vi "Main.vi"(11 "Module Admin":refnum<class "Delacor_lib_QMH_Module Admin.lvclass">) -> ()   [LabVIEW 2021, in "Master.lvlib"]
doc: "This template is based off of the Queued Message Handler design pattern and the Queued Message Handler project template that ships with LabVIEW.\n\nThe main difference is that the queue is private to this module and communication between modules is performed via Broadcast and Request events.\n\nRequest events are wrapped in public API methods and are handled in the Event Handling Loop (EHL) of this VI. Any module can register for Broadcast events sent by this module. The EHL generates messages based on user interface actions.\n\nThe Message Handling Loop (MHL) processes messages generated by the EHL, or by other messages. The messages are string values, so new messages can be added easily to the Message Cases case structure in the MHL. Each message cluster can also provide an optional value for Message Data, which is a variant that can be converted to whatever message-specific data is required.\n_____\nBased on DQMH Project Template 6.1.0.94.\n\n<b>Note:</b> This VI was modified by the <b>Validate DQMH Module</b> tool to add a 'Panel Hidden' status updated broadcast to the Panel Close? event when External Launch = TRUE.\n\n<b>Note:</b> This VI was modified by the <b>Validate DQMH Module</b> tool to add a call to the Error Reported VI at the end of the 'Exit' MHL frame.\n\n<b>Note:</b> This VI was modified by the <b>Validate DQMH Module</b> tool to wrap the FP.Open method in the module close code with a Conditional Disable Structure so it does not execute when the Main VI is running as a built EXE."
uses:
  Master.lvlib
  <vilib>/Delacor/Delacor QMH/Libraries/Module Admin_class/Delacor_lib_QMH_Module Admin.lvclass
  Custom/class Master/Master.lvclass
  <vilib>/Delacor/Delacor QMH/Libraries/Message Queue_class/Delacor_lib_QMH_Message Queue.lvclass/Delacor_lib_QMH_Message Queue.ctl
  Stop Argument--cluster.ctl
  <vilib>/Delacor/Delacor QMH/Libraries/Module Admin_class/Delacor_lib_QMH_Module Admin.lvclass/Delacor_lib_QMH_Module Admin.ctl
  Slave Stop Argument--cluster.ctl
  <vilib>/Utility/miscctls.llb/LVPointTypeDef.ctl
  Slave Launch Argument--cluster.ctl
  <vilib>/Delacor/Delacor QMH/Libraries/Message Queue_class/Delacor_lib_QMH_Enqueue Message (Single).vi
  <vilib>/Delacor/Delacor QMH/Libraries/Module Admin_class/Delacor_lib_QMH_Get External Launch.vi
  <vilib>/Utility/error.llb/Error Cluster From Error Code.vi
  <vilib>/ErrorRing/Error Ring.xnode
  <vilib>/Delacor/Delacor QMH/Libraries/Message Queue_class/Delacor_lib_QMH_Message Queue.lvclass
  Slave/Slave.lvlib
panel:
  in  "Slaves":i32=2
  in  "Launch Array":bool
  in  "Show Hide":bool
  out "Slave Launched":i32
  out "Slave Init":i32
  out "Slave Init?":bool
  in  "Show Slave":bool
  out "Err Module ID":i32
  out "Additional Information":string
  out "Slaves Error":errorcluster
  in  "Module ID":i32
  out "Slave IDs":i32[](array[numeric])
  in  "Stop Slave":bool
  in  "Launch Slave":bool
  out "Title":string
  out "error out":errorcluster
  out "Status":string
  in  "Simulate MHL Error":bool
  in  "Simulate EHL Error":bool
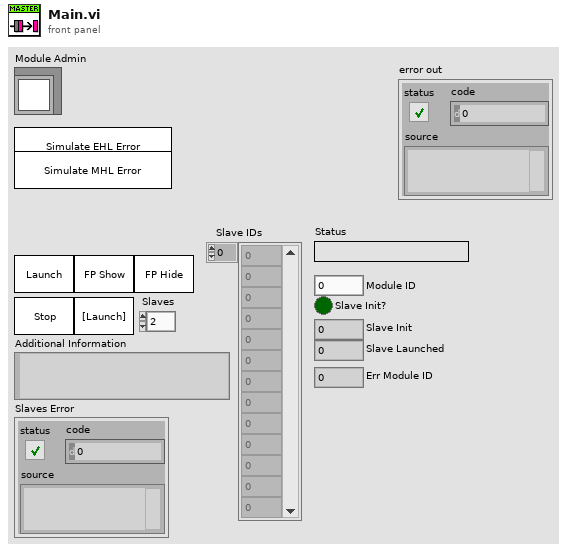
[diagram p1: front panel]
types:
  T1 = typedef "Master.lvlib/Request Events--cluster.ctl" = cluster{"Stop Module":refnum<user-event>, "Show Panel":refnum<user-event>, "Hide Panel":refnum<user-event>, "Get Module Execution Status":refnum<user-event>, "Show Diagram":refnum<user-event>, "Slave Launch":refnum<user-event>, "Slave Stop":refnum<user-event>}
  T2 = typedef "Slave.lvlib/Broadcast Events--cluster.ctl" = cluster{"Module Did Init":refnum<user-event>, "Status Updated":refnum<user-event>, "Error Reported":refnum<user-event>, "Module Did Stop":refnum<user-event>, "Update Module Execution Status":refnum<user-event>}
  T3 = enum32{"invalid lock state", "Not Locked", "Locked (No Password)", "Password-protected"}
  T4 = typedef "Master.lvlib/Stop Argument--cluster.ctl" = cluster{"Origin":string, "Exit via Stop Module Req?":bool, "Wait for Module to stop?":bool}
  T5 = typedef "Master.lvlib/Slave Stop Argument--cluster.ctl" = cluster{"Module ID":i32}
  T6 = typedef "LVPointTypeDef.ctl" = cluster{"Horizontal":i16, "Vertical":i16}
  T7 = enum32{"Invalid", "Standard", "Closed", "Hidden", "Minimized", "Maximized"}
  T8 = typedef "Master.lvlib/Slave Launch Argument--cluster.ctl" = cluster{"ModuleID":i32}
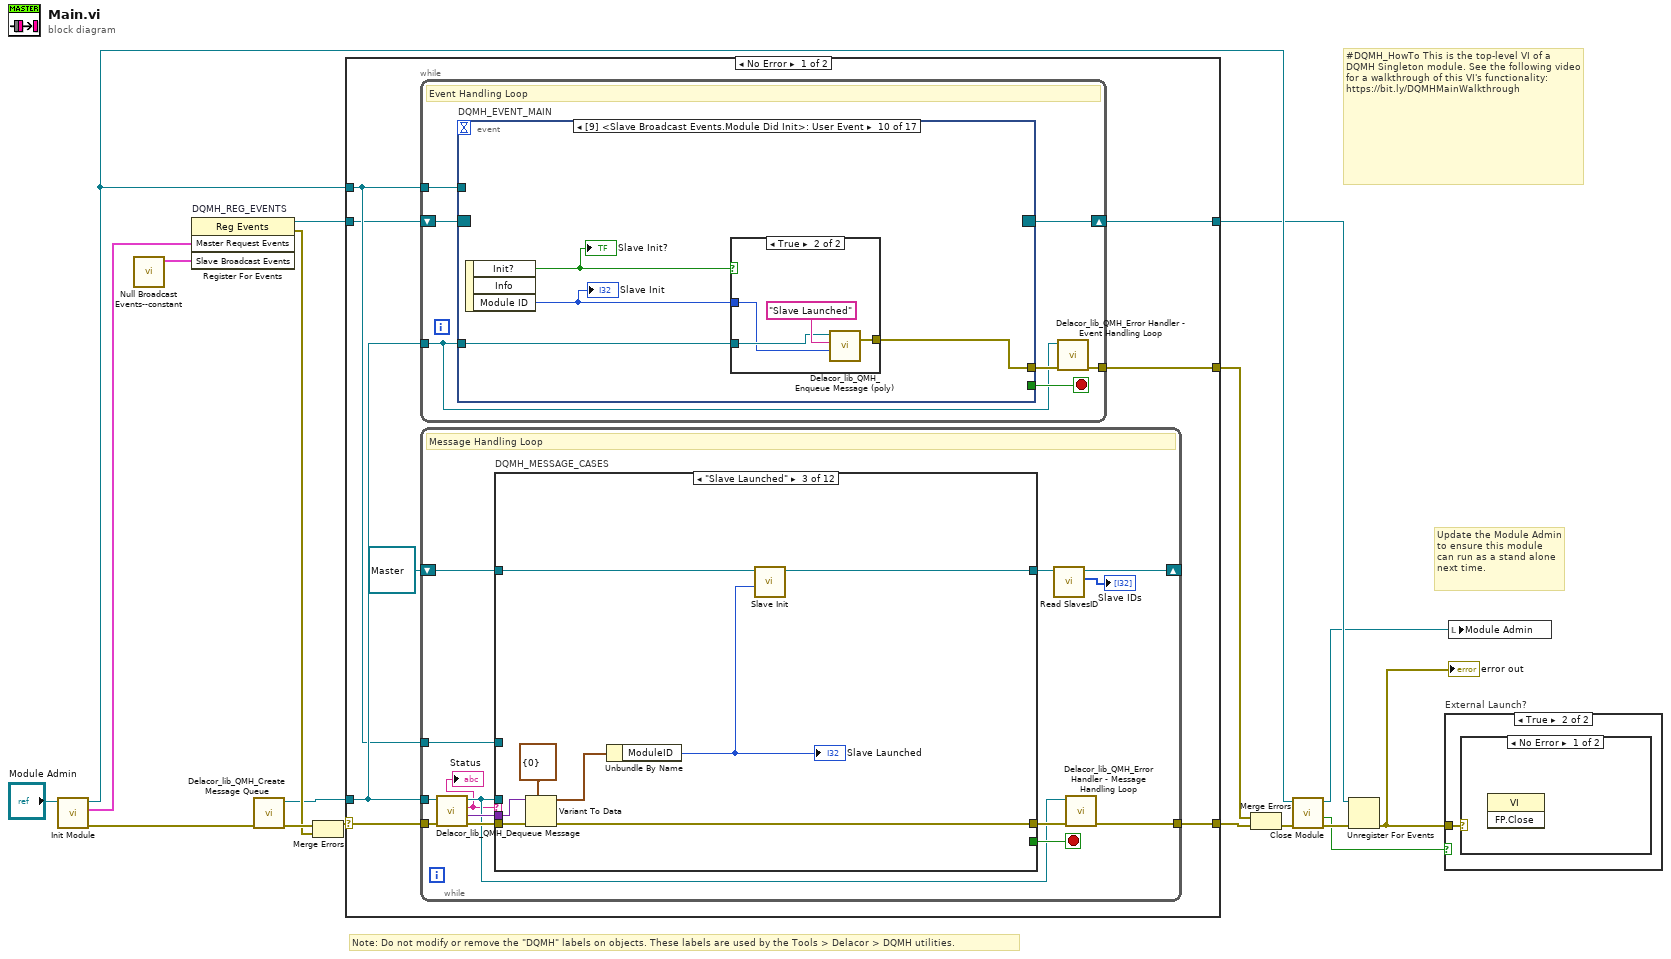
[diagram p0: block diagram]
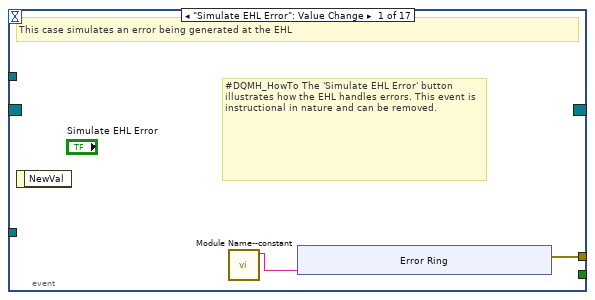
[diagram p2: hidden frame]
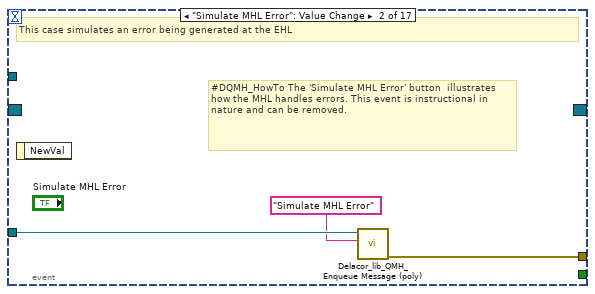
[diagram p3: hidden frame]
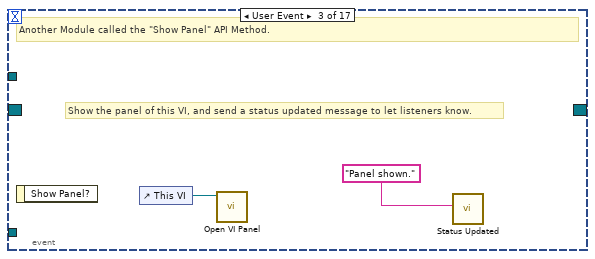
[diagram p4: hidden frame]
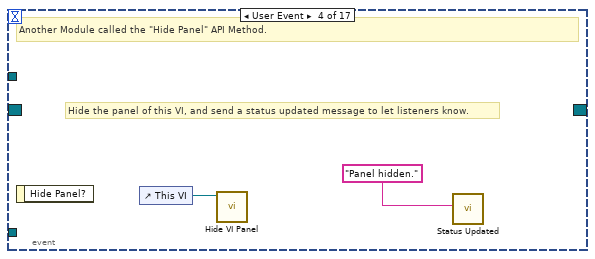
[diagram p5: hidden frame]
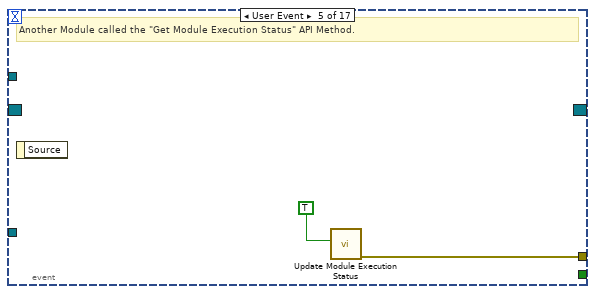
[diagram p6: hidden frame]
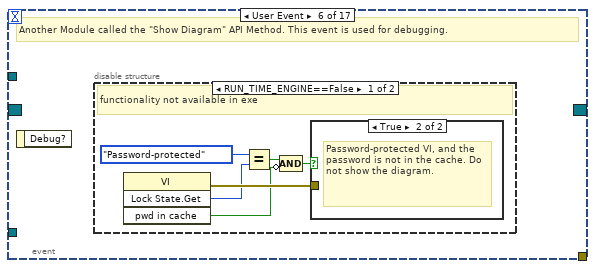
[diagram p7: hidden frame]
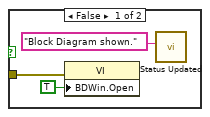
[diagram p8: hidden frame]
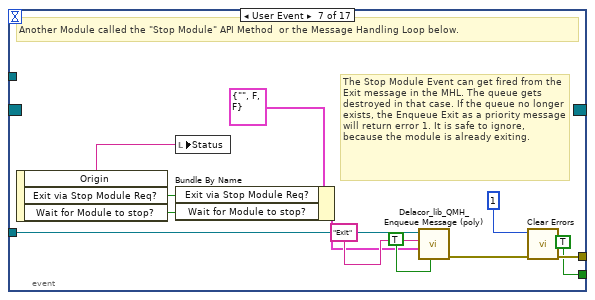
[diagram p10: hidden frame]
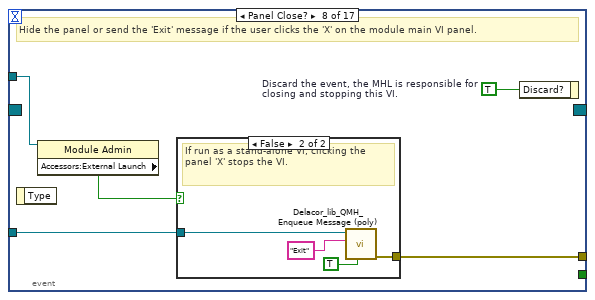
[diagram p11: hidden frame]
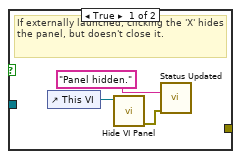
[diagram p12: hidden frame]
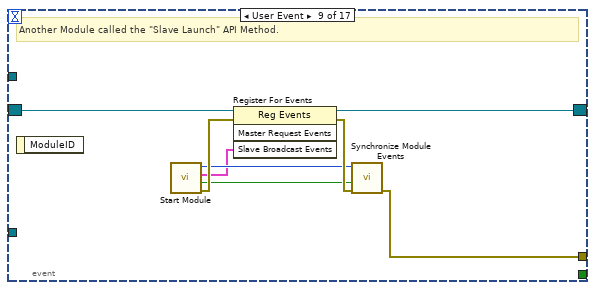
[diagram p13: hidden frame]
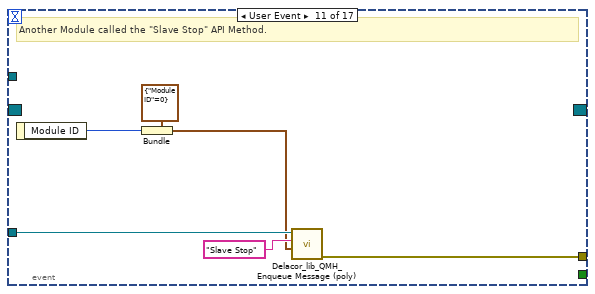
[diagram p15: hidden frame]
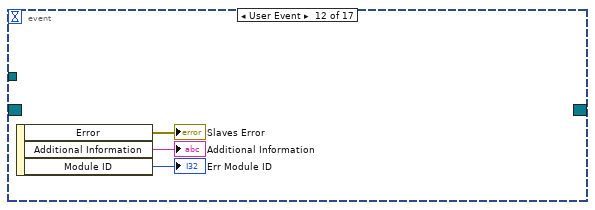
[diagram p16: hidden frame]
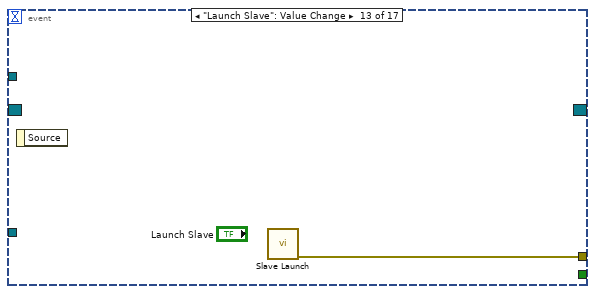
[diagram p17: hidden frame]
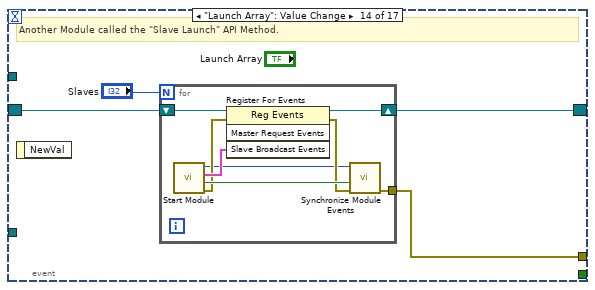
[diagram p18: hidden frame]
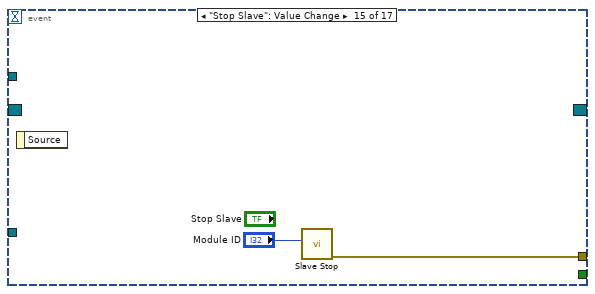
[diagram p19: hidden frame]
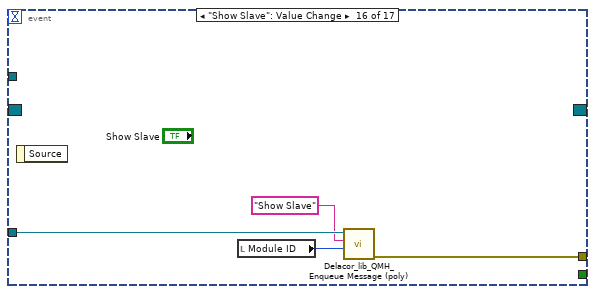
[diagram p20: hidden frame]
diagram:
  # "#DQMH_HowTo This is the top-level VI of a DQMH Singleton module. See the following video for a walkthrough of this VI's functionality: https://bit.ly/DQMHMainWalkthrough"
  # "Note: Do not modify or remove the \"DQMH\" labels on objects. These labels are used by the Tools > Delacor > DQMH utilities."
  # "Update the Module Admin to ensure this module can run as a stand alone next time."
  n1 = call "Init Module.vi"("Singleton Module Admin in"="Module Admin") -> ("error out"=w17:errorcluster, "Master Request Events"=w6:T1, "Singleton Module Admin out"=w9:refnum<class "Delacor_lib_QMH_Module Admin.lvclass">)  [unwired: 8 in]
  n2 = call "Null Broadcast Events--constant.vi"() -> ("Slave Broadcast Events"=w1:T2)  [unwired: 11 in]
  n3 = register-events "DQMH_REG_EVENTS"(w6, w1) -> (reference out=w7:refnum<event-registration>, error out=w10:errorcluster)  [unwired: 2 in]
  n4 = call <vilib>:"Delacor_lib_QMH_Create Message Queue.vi"("error in"=w17) -> ("error out"=w12:errorcluster, "Message Queue"=w5:refnum<class "Delacor_lib_QMH_Message Queue.lvclass">)  [unwired: 9 in]
  n5 = Merge Errors(w12, w10) -> (w11:errorcluster)
  n6 = case shown="No Error" w11 {
    selector: w11 -> [w24 w267]
    tunnel: [w26 w266] -> w18
    tunnel: [w23 w272] -> w8
    tunnel: w7 -> [w19 w272]
    tunnel: w5 -> [w21 w265]
    tunnel: [w25 _] -> w15
    tunnel: w9 -> [w20 w268]
    frame No Error {
      n7 = while {
        tunnel: w21 -> [w27]
        shift-right: [w30] -> w23
        shift-left: w19 -> [w31]
        tunnel: [w32] -> w25
        tunnel: w20 -> [w28]
        stop <- w29 stop-if-true
        # "Event Handling Loop"
        n8 = event "DQMH_EVENT_MAIN" shown="[9] <Slave Broadcast Events.Module Did Init>: User Event" {
          selector: w31 -> [_ _ _ _ _ _ _ _ w92 _ _ _ _ w114 _ _ _]
          dyn-events: [_ _ _ _ _ _ _ _ w91 _ _ _ _ w113 _ _ _] -> w30
          timeout: _ -> [_ _ _ _ _ _ _ _ _ _ _ _ _ _ _ _ _]
          tunnel: [_ _ _ _ _ _ TRUE ("Discard?") _ _ _ _ _ _ _ _ _ _] -> w29
          tunnel: w27 -> [_ w44 _ _ _ _ w68 w75 _ w93 w106 _ _ _ _ w127 w130]
          tunnel: [w35 w45 _ _ w51 _ w71 w77 w90 w94 w101 _ w110 w112 w124 w128 w129] -> w33
          tunnel: w28 -> [_ _ _ _ _ _ _ w74 _ _ _ _ _ _ _ _ _]
          event "Simulate EHL Error": Value Change {
            # "#DQMH_HowTo The 'Simulate EHL Error' button  illustrates how the EHL handles errors. This event is instructional in nature and can be removed."
            # "This case simulates an error being generated at the EHL"
            n9 = event-data() -> ()  [unwired: 1 in, 1 out]
            n10 = call "Module Name--constant.vi"() -> ("Module Name"=w34:string)  [unwired: 11 in]
            n11 = xnode ("Error Ring")("parameter 0"=w34) -> ("error out"=w35:errorcluster)
          }
          event "Simulate MHL Error": Value Change {
            # "#DQMH_HowTo The 'Simulate MHL Error' button  illustrates how the MHL handles errors. This event is instructional in nature and can be removed."
            # "This case simulates an error being generated at the EHL"
            n12 = event-data() -> ()  [unwired: 1 in, 1 out]
            n13 = call-poly <vilib>:"Delacor_lib_QMH_Enqueue Message (poly).vi"("Message"="Simulate MHL Error", "Message Queue in"=w44) -> ("error out"=w45:errorcluster)  [unwired: 8 in, 1 out]
          }
          event User Event {
            # "Show the panel of this VI, and send a status updated message to let listeners know."
            # "Another Module called the \"Show Panel\" API Method."
            n14 = event-data() -> ()  [unwired: 1 in, 1 out]
            n15 = control-ref of="This VI"() -> (w47:refnum<vi>)
            n16 = call "Open VI Panel.vi"("VI"=w47) -> ()  [unwired: 10 in, 1 out]
            n17 = call "Status Updated.vi"("Status"="Panel shown." ("format string")) -> ()  [unwired: 10 in, 1 out]
          }
          event User Event {
            # "Hide the panel of this VI, and send a status updated message to let listeners know."
            # "Another Module called the \"Hide Panel\" API Method."
            n18 = event-data() -> ()  [unwired: 1 in, 1 out]
            n19 = control-ref of="This VI"() -> (w49:refnum<vi>)
            n20 = call "Hide VI Panel.vi"("VI"=w49) -> ()  [unwired: 10 in, 1 out]
            n21 = call "Status Updated.vi"("Status"="Panel hidden." ("format string")) -> ()  [unwired: 10 in, 1 out]
          }
          event User Event {
            # "Another Module called the \"Get Module Execution Status\" API Method."
            n22 = event-data() -> ()  [unwired: 1 in, 1 out]
            n23 = call "Update Module Execution Status.vi"("Running?"=TRUE) -> ("error out"=w51:errorcluster)  [unwired: 10 in]
          }
          event User Event {
            # "Another Module called the \"Show Diagram\" API Method. This event is used for debugging."
            n24 = event-data() -> ()  [unwired: 1 in, 1 out]
            n25 = disable-structure "Conditional Disable Structure" shown="RUN_TIME_ENGINE==False" {
              frame condition #0 (active) {
                # "functionality not available in exe"
                n26 = invoke on="Invoke Node" class="VI" method="Lock State.Get"() -> (error out=w57:errorcluster, "Get Lock State"=w56:T3, "pwd in cache"=w53:bool)  [unwired: 4 in, 1 out]
                n27 = Equal?(x=T3."Password-protected", y=w56) -> (x = y?=w54:bool)
                n28 = Compound Arithmetic op=AND(w54, invert w53) -> (w52:bool)
                n29 = case shown="True" w52 {
                  tunnel: w57 -> [w60 _]
                  frame False {
                    n30 = property on="Property Node" class="VI"(error in=w60, "BDWin.Open"=TRUE ("Block Diagram Window:Open")) -> ()  [unwired: 1 in, 2 out]
                    n31 = call "Status Updated.vi"("Status"="Block Diagram shown." ("format string")) -> ()  [unwired: 10 in, 1 out]
                  }
                  frame True {
                    # "Password-protected VI, and the password is not in the cache. Do not show the diagram."
                  }
                }
              }
              frame condition #1 {
              }
            }
          }
          event User Event {
            # "The Stop Module Event can get fired from the Exit message in the MHL. The queue gets destroyed in that case. If the queue no longer exists, the Enqueue Exit as a priority message will return error 1. It is safe to ignore, because the module is already exiting."
            # "Another Module called the \"Stop Module\" API Method  or the Message Handling Loop below."
            n32 = event-data() -> ("Origin"=w67:string, "Exit via Stop Module Req?"=w63:bool, "Wait for Module to stop?"=w62:bool)  [unwired: 1 in]
            n33 = local write "Status"(w67) -> ()
            n34 = Bundle By Name(cluster=T4 {"Origin"="", "Exit via Stop Module Req?"=FALSE, "Wait for Module to stop?"=FALSE} ("Stop Argument"), "Exit via Stop Module Req?"=w63, "Wait for Module to stop?"=w62) -> (w61:T4)
            n35 = call-poly <vilib>:"Delacor_lib_QMH_Enqueue Message (poly).vi"("Priority Message? (F)"=TRUE, "Message Data"=w61, "Message"="Exit", "Message Queue in"=w68) -> ("error out"=w72:errorcluster)  [unwired: 6 in, 1 out]
            n36 = call <vilib>:"Clear Errors.vi"("error in (no error)"=w72, "specific error code to clear (0: all)"=1) -> ("error out"=w71:errorcluster)  [unwired: 4 in, 1 out]
          }
          event Panel Close? {
            w76 = TRUE  # Discard the event, the MHL is responsible for closing and stopping this VI.
            # "Hide the panel or send the 'Exit' message if the user clicks the 'X' on the module main VI panel."
            n37 = event-data() -> ()  [unwired: 1 in, 1 out]
            n38 = property on="Property Node" class="Module Admin"(reference=w74) -> ("Accessors:External Launch"=w73:bool)  [unwired: 1 in, 2 out]
            n39 = case shown="False" w73 {
              tunnel: w75 -> [_ w83]
              tunnel: [_ w84] -> w77
              frame True {
                # "If externally launched, clicking the 'X' hides the panel, but doesn't close it."
                n40 = control-ref of="This VI"() -> (w80:refnum<vi>)
                n41 = call "Hide VI Panel.vi"("VI"=w80) -> ("error out"=w78:errorcluster)  [unwired: 10 in]
                n42 = call "Status Updated.vi"("error in (no error)"=w78, "Status"="Panel hidden.") -> ()  [unwired: 9 in, 1 out]
              }
              frame False {
                # "If run as a stand-alone VI, clicking the panel 'X' stops the VI."
                n43 = call-poly <vilib>:"Delacor_lib_QMH_Enqueue Message (poly).vi"("Priority Message? (F)"=TRUE, "Message"="Exit", "Message Queue in"=w83) -> ("error out"=w84:errorcluster)  [unwired: 7 in, 1 out]
              }
            }
            n44 = event-data ("Event Filter Node")("Discard?"=w76) -> ()  [unwired: 1 in, 1 out]
          }
          event User Event {
            # "Another Module called the \"Slave Launch\" API Method."
            n45 = event-data() -> ()  [unwired: 1 in, 1 out]
            n46 = call "Start Module.vi"() -> ("error out"=w89:errorcluster, "Wait for Event Sync?"=w85:bool, "Slave Broadcast Events"=w86:T2, "Module ID"=w87:i32)  [unwired: 8 in]
            n47 = register-events(reference=w92, error in=w89, w86) -> (reference out=w91:refnum<event-registration>, error out=w88:errorcluster)  [unwired: 1 in]
            n48 = call "Synchronize Module Events.vi"("error in"=w88, "Wait for Event Sync?"=w85, "Module ID in"=w87) -> ("error out"=w90:errorcluster)  [unwired: 7 in, 1 out]
          }
          event User Event {
            n49 = event-data() -> ("Init?"=w96:bool, "Module ID"=w95:i32)  [unwired: 1 in, 1 out]
            "Slave Init?" <- w96
            "Slave Init" <- w95
            n50 = case shown="True" w96 {
              tunnel: [_ w98] -> w94
              tunnel: w93 -> [_ w99]
              tunnel: w95 -> [_ w97]
              frame False {
              }
              frame True {
                n51 = call-poly <vilib>:"Delacor_lib_QMH_Enqueue Message (poly).vi"("Message Data"=w97, "Message"="Slave Launched", "Message Queue in"=w99) -> ("error out"=w98:errorcluster)  [unwired: 7 in, 1 out]
              }
            }
          }
          event User Event {
            # "Another Module called the \"Slave Stop\" API Method."
            n52 = event-data() -> ("Module ID"=w102:i32)  [unwired: 1 in]
            n53 = Bundle(cluster=T5 {"Module ID"=0} ("Slave Stop Argument"), "Module ID"=w102) -> (w103:T5)
            n54 = call-poly <vilib>:"Delacor_lib_QMH_Enqueue Message (poly).vi"("Message Data"=w103, "Message"="Slave Stop", "Message Queue in"=w106) -> ("error out"=w101:errorcluster)  [unwired: 7 in, 1 out]
          }
          event User Event {
            n55 = event-data() -> ("Error"=→"Slaves Error":errorcluster, "Additional Information"=→"Additional Information":string, "Module ID"=→"Err Module ID":i32)  [unwired: 1 in]
          }
          event "Launch Slave": Value Change {
            n56 = event-data() -> ()  [unwired: 1 in, 1 out]
            n57 = call "Slave Launch.vi"() -> ("error out"=w110:errorcluster)  [unwired: 11 in]
          }
          event "Launch Array": Value Change {
            # "Another Module called the \"Slave Launch\" API Method."
            n58 = event-data() -> ()  [unwired: 1 in, 1 out]
            n59 = for {
              N: "Slaves" -> [_]
              tunnel: [w120] -> w112
              shift-right: [w121] -> w113
              shift-left: w114 -> [w122]
              n60 = call "Start Module.vi"() -> ("error out"=w117:errorcluster, "Wait for Event Sync?"=w118:bool, "Slave Broadcast Events"=w119:T2, "Module ID"=w115:i32)  [unwired: 8 in]
              n61 = register-events(reference=w122, error in=w117, w119) -> (reference out=w121:refnum<event-registration>, error out=w116:errorcluster)  [unwired: 1 in]
              n62 = call "Synchronize Module Events.vi"("error in"=w116, "Wait for Event Sync?"=w118, "Module ID in"=w115) -> ("error out"=w120:errorcluster)  [unwired: 7 in, 1 out]
            }
          }
          event "Stop Slave": Value Change {
            n63 = event-data() -> ()  [unwired: 1 in, 1 out]
            n64 = call "Slave Stop.vi"("Module ID"="Module ID") -> ("error out"=w124:errorcluster)  [unwired: 10 in]
          }
          event "Show Slave": Value Change {
            n65 = event-data() -> ()  [unwired: 1 in, 1 out]
            n66 = local read "Module ID"() -> (w125:i32)
            n67 = call-poly <vilib>:"Delacor_lib_QMH_Enqueue Message (poly).vi"("Message Data"=w125, "Message"="Show Slave", "Message Queue in"=w127) -> ("error out"=w128:errorcluster)  [unwired: 7 in, 1 out]
          }
          event "Show Hide": Value Change {
            n68 = event-data() -> ()  [unwired: 1 in, 1 out]
            n69 = local read "Module ID"() -> (w131:i32)
            n70 = call-poly <vilib>:"Delacor_lib_QMH_Enqueue Message (poly).vi"("Message Data"=w131, "Message"="Hide Slave", "Message Queue in"=w130) -> ("error out"=w129:errorcluster)  [unwired: 7 in, 1 out]
          }
        }
        n71 = call-dynamic "Delacor_lib_QMH_Error Handler - Event Handling Loop.vi"("error in"=w33, "Message Queue in"=w27) -> ("dup error in"=w32:errorcluster)  [unwired: 8 in, 1 out]
      }
      n72 = while {
        tunnel: w21 -> [w139]
        shift-right: [w135] -> _
        shift-left: refnum<class "Master.lvclass"> refnum ("Data Cluster") -> [w142]
        tunnel: w24 -> [w145]
        tunnel: [w143] -> w26
        tunnel: w20 -> [w137]
        stop <- w141 stop-if-true
        # "Message Handling Loop"
        n73 = call-dynamic "Delacor_lib_QMH_Dequeue Message.vi"("error in"=w145, "Message Queue in"=w139) -> ("error out"=w144:errorcluster, "Message Data"=w140:variant, "Message"=w136:string, "Message Queue out"=w138:refnum<class "Delacor_lib_QMH_Message Queue.lvclass">)  [unwired: 6 in]
        "Status" <- w136
        n74 = case "DQMH_MESSAGE_CASES" shown="\"Slave Launched\"" w136 {
          selector: w136 -> [_ _ _ _ _ _ _ _ _ _ _ w252]
          tunnel: w138 -> [_ _ _ _ _ _ _ _ _ w220 w244 _]
          tunnel: w144 -> [w163 w166 w174 w184 w192 w200 w203 w205 w210 w227 w250 w254]
          tunnel: [w161 w166 w171 w176 w187 w195 w202 w205 w209 w223 w247 w255] -> w146
          tunnel: w142 -> [w153 w165 w172 w179 w191 w199 w201 w204 w207 w222 w243 w253]
          tunnel: [w147 w165 w169 w178 w191 w199 w201 w204 w207 w222 w235 w253] -> w133
          tunnel: [_ _ _ _ _ _ _ _ _ _ w242 _] -> w141
          tunnel: w140 -> [_ _ w173 w182 w190 w198 _ _ _ w221 w241 _]
          tunnel: w137 -> [w154 _ _ _ _ _ _ _ _ w219 w236 _]
          frame "Initialize" {
            # "Initialize - Any operation that needs to be done before the module can receive messages. Synchronize Caller Events.vi will inform Start Module.vi that the module has launched and is ready to receive messages. Module Did Init.vi will broadcast that the module initialized."
            n75 = call "Synchronize Caller Events.vi"("error in (no error)"=w163, "Singleton Module Admin in"=w154) -> ("error out"=w162:errorcluster, "Singleton Module Admin out"=w150:refnum<class "Delacor_lib_QMH_Module Admin.lvclass">)  [unwired: 8 in]
            n76 = property on="Pane" class="Pane"("Origin"=T6 {"Horizontal"=0, "Vertical"=0}) -> ()  [unwired: 2 in, 2 out]
            n77 = property on="Property Node" class="Module Admin"(reference=w150) -> ("Accessors:External Launch"=w158:bool)  [unwired: 1 in, 2 out]
            n78 = call "Module Name--constant.vi"() -> ("Module Name"=w148:string)  [unwired: 11 in]
            "Title" <- w148
            n79 = property on="Property Node" class="VI"("Front Panel.Title"=w148) -> (reference out=w160:refnum<vi>, error out=w164:errorcluster)  [unwired: 2 in]
            n80 = Select(t=T7."Hidden" ("State"), s=w158, f=T7."Standard" ("State")) -> (s? t:f=w155:T7)
            n81 = invoke on="Invoke Node" class="VI" method="FP.Open"(reference=w160, error in=w164, "State"=w155) -> (reference out=w159:refnum<vi>)  [unwired: 2 in, 4 out]
            n82 = call "Init Vars.vi"("Master in"=w153) -> ("Master out"=w147:refnum<class "Master.lvclass">)  [unwired: 9 in, 1 out]
            n83 = call "FP Position.vi"("This VI"=w159) -> ()  [unwired: 11 in]
            n84 = call "Module Name--constant.vi"() -> ("Module Name"=w151:string)  [unwired: 11 in]
            n85 = call "Module Did Init.vi"("error in (no error)"=w162, "Initialized?"=TRUE, "Origin"=w151) -> ("error out"=w161:errorcluster)  [unwired: 8 in]
          }
          frame "---Module Specific---" {
            # "Separator -- The following cases handle messages specific to this Module."
          }
          frame "Slave Launched" {
            n86 = Variant To Data(error in=w174, type=T8 {"ModuleID"=0} ("Slave Launch Argument"), Variant=w173) -> (data=w170:T8, error out=w171:errorcluster)
            n87 = Unbundle By Name(w170) -> ("ModuleID"=w167:i32)
            "Slave Launched" <- w167
            n88 = call "Slave Init.vi"("ID"=w167, "Master in"=w172) -> ("Master out"=w169:refnum<class "Master.lvclass">)  [unwired: 8 in, 1 out]
          }
          frame "Slave Stop" {
            n89 = Variant To Data(error in=w184, type=T5 {"Module ID"=0} ("Slave Stop Argument"), Variant=w182) -> (data=w180:T5, error out=w183:errorcluster)
            n90 = Unbundle By Name(w180) -> ("Module ID"=w177:i32)
            n91 = call "Slave Stop.vi"("ID"=w177, "Master in"=w179) -> ("error out"=w175:errorcluster, "Master out"=w178:refnum<class "Master.lvclass">)  [unwired: 8 in]
            n92 = Merge Errors(w183, w175) -> (w176:errorcluster)
          }
          frame "Show Slave" {
            n93 = Variant To Data(error in=w192, type=-1 ("Module ID"), Variant=w190) -> (data=w188:i32, error out=w186:errorcluster)
            n94 = call "Show Panel.vi"("Module ID"=w188) -> ("error out"=w185:errorcluster)  [unwired: 10 in]
            n95 = Merge Errors(w186, w185) -> (w187:errorcluster)
          }
          frame "Hide Slave" {
            n96 = Variant To Data(error in=w200, type=-1 ("Module ID"), Variant=w198) -> (data=w196:i32, error out=w194:errorcluster)
            n97 = call "Hide Panel.vi"("Module ID"=w196) -> ("error out"=w193:errorcluster)  [unwired: 10 in]
            n98 = Merge Errors(w194, w193) -> (w195:errorcluster)
          }
          frame "---Copy This Frame---" {
            # "Duplicate this frame when creating new messages.  Change this comment in the duplicated frame to describe this message."
            n99 = Merge Errors(w203) -> (w202:errorcluster)
          }
          frame "---Exit and Error Handling---" {
            # "Separator - The following cases handle errors and exit messages."
          }
          frame "Simulate MHL Error" {
            # "#DQMH_HowTo The 'Simulate MHL Error' button  illustrates how the MHL handles errors. This event is instructional in nature and can be removed."
            # "Simulate an error occurring at the MHL"
            n100 = call "Module Name--constant.vi"() -> ("Module Name"=w206:string)  [unwired: 11 in]
            n101 = xnode ("Error Ring")("parameter 0"=w206) -> ("error out"=w208:errorcluster)
            n102 = Merge Errors(w210, w208) -> (w209:errorcluster)
          }
          frame "Error" {
            # "#CodeRecommended - If you ever change the name of this \"Error\" message, you'll need to update the name in the Check Loop Error.vi as well."
            # "#CodeRecommended - If the module is running in standalone mode (External Launch = FALSE), this code will pop up an error dialog and call the 'Exit' message if an error occurs. Add more fine-grained error handling here."
            # "Error - Check the error message data and respond accordingly. This message is sent by the \"Error Handler\" VIs at the end of each loop in this application."
            n103 = property on="Property Node" class="Module Admin"(reference=w219) -> ("Accessors:External Launch"=w218:bool)  [unwired: 1 in, 2 out]
            n104 = Variant To Data(error in=w227, type=errorcluster {"status"=FALSE, "code"=0, "source"=""} ("error constant"), Variant=w221) -> (data=w228:errorcluster, error out=w225:errorcluster)
            n105 = call "Error Reported.vi"("Error"=w228) -> ()  [unwired: 10 in, 1 out]
            n106 = case shown="False" w218 {
              tunnel: [w233 _] -> w224
              tunnel: w220 -> [w231 _]
              tunnel: w228 -> [w232 _]
              frame False {
                # "If the module is running standalone, then pop up an error dialog and call the \"Exit\" message."
                n107 = call <vilib>:"Simple Error Handler.vi"("error in (no error)"=w232) -> ()  [unwired: 4 in, 5 out]
                n108 = call-poly <vilib>:"Delacor_lib_QMH_Enqueue Message (poly).vi"("Priority Message? (F)"=TRUE, "Message"="Exit", "Message Queue in"=w231) -> ("error out"=w233:errorcluster)  [unwired: 7 in, 1 out]
              }
              frame True {
                # "If the module was launched externally, calling the Error Reported broadcast VI is the only action performed by the \"Error\" message. The module's caller can then process the error appropriately."
              }
            }
            n109 = Merge Errors(w225, w224) -> (w223:errorcluster)
            n110 = local write "error out"(w223) -> ()
          }
          frame "Exit" {
            w240 = 91  # 91: not all Exit messages will have an argument
            w242 = TRUE  # Stop the VI
            # "Release the message queue reference"
            # "Exit - Exit the application."
            n111 = control-ref of="This VI"() -> (w237:refnum<vi>)
            n112 = Variant To Data(error in=w250, type=T4 {"Origin"="", "Exit via Stop Module Req?"=FALSE, "Wait for Module to stop?"=FALSE} ("Stop Argument"), Variant=w241) -> (data=w238:T4, error out=w246:errorcluster)
            n113 = call "Handle Exit.vi"("Stop Argument"=w238, "Admin in"=w236, "VI reference"=w237) -> ("error out"=w245:errorcluster)  [unwired: 7 in, 1 out]
            n114 = call <vilib>:"Clear Errors.vi"("error in (no error)"=w246, "specific error code to clear (0: all)"=w240) -> ("error out"=w249:errorcluster)  [unwired: 4 in, 1 out]
            n115 = call-dynamic "Delacor_lib_QMH_Release Message Queue.vi"("error in"=w249, "Message Queue"=w244) -> ("error out"=w248:errorcluster)  [unwired: 9 in]
            n116 = call "DeInit.vi"("Master in"=w243) -> ("error out"=w234:errorcluster, "Master out"=w235:refnum<class "Master.lvclass">)  [unwired: 9 in]
            n117 = Merge Errors(w248, w245, w234) -> (w247:errorcluster)
            n118 = call "Error Reported.vi"("Error"=w247) -> ()  [unwired: 10 in, 1 out]
          }
          frame Default {
            # "'Default' case only runs if there is a message that isn't defined in any of the other cases.  Output a programming error."
            n119 = call "Module Name--constant.vi"() -> ("Module Name"=w251:string)  [unwired: 11 in]
            n120 = xnode ("Error Ring")("parameter 0"=w252, "parameter 1"=w251) -> ("error out"=w256:errorcluster)
            n121 = Merge Errors(w254, w256) -> (w255:errorcluster)
          }
        }
        n122 = call-dynamic "Read SlavesID.vi"("Master in"=w133) -> ("SlavesID"=→"Slave IDs":i32[], "Master out"=w135:refnum<class "Master.lvclass">)  [unwired: 8 in, 1 out]
        n123 = call-dynamic "Delacor_lib_QMH_Error Handler - Message Handling Loop.vi"("error in"=w146, "Message Queue in"=w138) -> ("dup error in"=w143:errorcluster)  [unwired: 8 in, 1 out]
      }
    }
    frame Error {
      # "Synchronize Caller Events.vi will inform Start Module.vi that the module has launched and will let the code calling Start Module.vi register for broadcasts and would permit the caller receive the broadcast that an error occurred at launch time."
      n124 = call-dynamic "Delacor_lib_QMH_Release Message Queue.vi"("error in"=w267, "Message Queue"=w265) -> ("error out"=w266:errorcluster)  [unwired: 9 in]
      n125 = call "Synchronize Caller Events.vi"("Singleton Module Admin in"=w268) -> ("error out"=w273:errorcluster)  [unwired: 9 in, 1 out]
      n126 = call "Module Name--constant.vi"() -> ("Module Name"=w271:string)  [unwired: 11 in]
      n127 = Format Into String(format string="An error occurred during initialization. %s is no longer running.", w271) -> (resulting string=w269:string)  [unwired: 2 in, 1 out]
      n128 = Merge Errors(w266, w273) -> (w274:errorcluster)
      n129 = call "Error Reported.vi"("Additional Information"=w269, "Error"=w274) -> ()  [unwired: 9 in, 1 out]
    }
  }
  n130 = Merge Errors(w15, w18) -> (w14:errorcluster)
  n131 = call "Close Module.vi"("error in (no error)"=w14, "Module Admin in"=w9) -> ("error out"=w16:errorcluster, "External Launch"=w2:bool, "Module Admin out"=w3:refnum<class "Delacor_lib_QMH_Module Admin.lvclass">)  [unwired: 7 in]
  n132 = Unregister For Events(event registration refnum=w8, error in=w16) -> (error out=w13:errorcluster)
  "error out" <- w13
  n133 = case "External Launch?" shown="True" w2 {
    tunnel: w13 -> [_ w275]
    frame False {
    }
    frame True {
      n134 = case shown="No Error" w275 {
        frame No Error {
          n135 = invoke on="Invoke Node" class="VI" method="FP.Close"() -> ()  [unwired: 3 in, 3 out]
        }
        frame Error {
          n136 = disable-structure shown="Default" {
            frame condition #0 (active) {
              n137 = invoke class="VI" method="FP.Open"("Activate"=TRUE ("Activate?")) -> ()  [unwired: 4 in, 5 out]
            }
            frame condition #1 {
              # "Don't show panel on error if running inside a built EXE."
            }
          }
        }
      }
    }
  }
  n138 = local write "Module Admin"(w3) -> ()
